vi "factorial function.vi"() -> ()   [LabVIEW 2023]
panel:
  in  "Numeric 3":i32
  out "Numeric 4":i32
  out "Numeric 2":i32
  in  "Numeric":i32
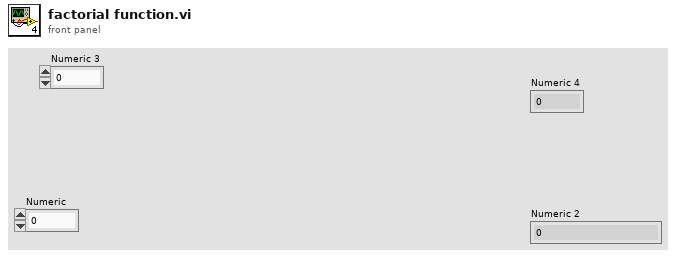
[diagram p1: front panel]
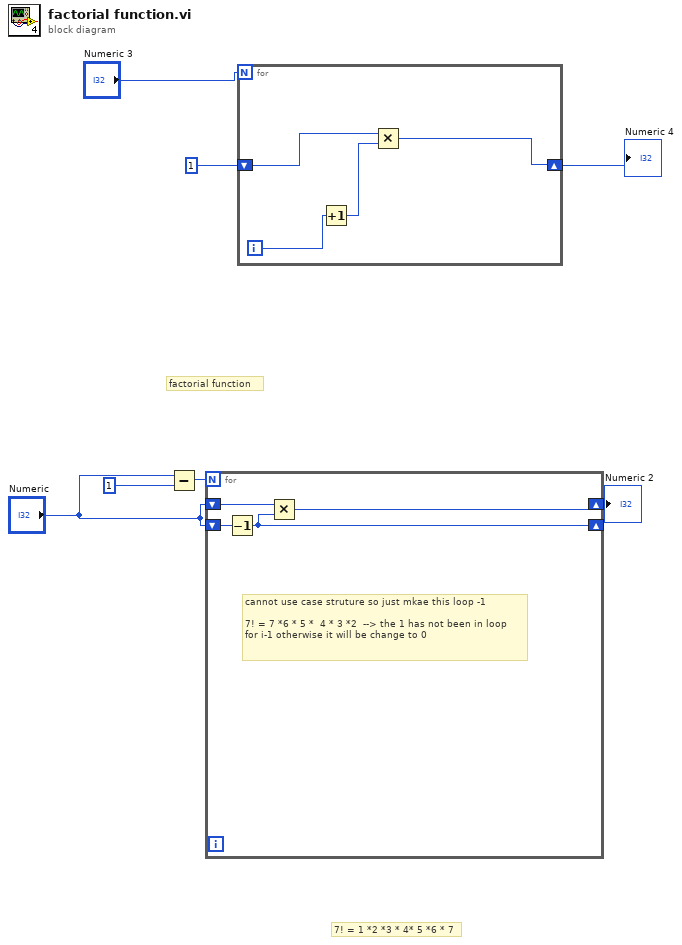
[diagram p0: block diagram]
diagram:
  # "7! = 1 *2 *3 * 4* 5 *6 * 7"
  # "factorial function"
  n1 = Subtract(x="Numeric", y=1) -> (x-y=w5:i32)
  n2 = for {
    N: w5 -> [_]
    shift-right: [w10] -> w7
    shift-left: "Numeric" -> [w9]
    shift-right: [w8] -> _
    shift-left: "Numeric" -> [w11]
    # "cannot use case struture so just mkae this loop -1 \n\n7! = 7 *6 * 5 *  4 * 3 *2  --> the 1 has not been in loop\nfor i-1 otherwise it will be change to 0"
    n3 = Decrement(x=w11) -> (x-1=w8:i32)
    n4 = Multiply(x=w9, y=w8) -> (x*y=w10:i32)
  }
  "Numeric 2" <- w7
  n5 = for {
    N: "Numeric 3" -> [_]
    shift-right: [w12] -> w1
    shift-left: 1 -> [w14]
    i -> [w15]
    n6 = Increment(x=w15) -> (x+1=w13:i32)
    n7 = Multiply(x=w14, y=w13) -> (x*y=w12:i32)
  }
  "Numeric 4" <- w1
